vi "AndorCamera.vi"() -> ()   [LabVIEW 2018, in "AndorOWN.lvlib"]
uses:
  AndorOWN.lvlib
  Andor SDK/AndorSDK.lvlib
  SOLA/LabVIEW 2015 Library (32bit)/LumencorDLL32/LumencorDLL32.lvlib
panel:
  out "speed out":sgl
  out "fastest speed out":sgl
  out "fastest index out":i32
  out "LETypeStr out":string
  in  "ComPort":i32=5
  out "Image":T1(plugin-control)
  out "Acq. Error Array":cluster{i32, string}[](array[cluster])
  in  "Set Temperature":i32=-20
  out "Acquisition Ready?":bool
  in  "Abort Acquisition":bool
  in  "Image Name":string="TestIMG"
  in  "Camera Messages":i32(listbox)=2
  in  "Acquire Image":bool
  out "kinetic out":sgl
  out "accumulate out":sgl
  out "exposure out":sgl
  in  "Exposure Time [ms]":sgl=50.0
  in  "stop":bool
  out "Cooling Message":cluster{i32, string}
  out "Camera Temperature":sgl
  out "temperature out":sgl
  out "mintemp out":i32
  out "maxtemp out":i32
  out "AmbientTemp out":sgl
  out "TargetTemp out":sgl
  out "SensorTemp out":sgl
  out "CoolerVolts out":sgl
  out "xpixels out":i32
  out "ypixels out":i32
  out "cameraHandle out":i32
  out "totalCameras out":i32
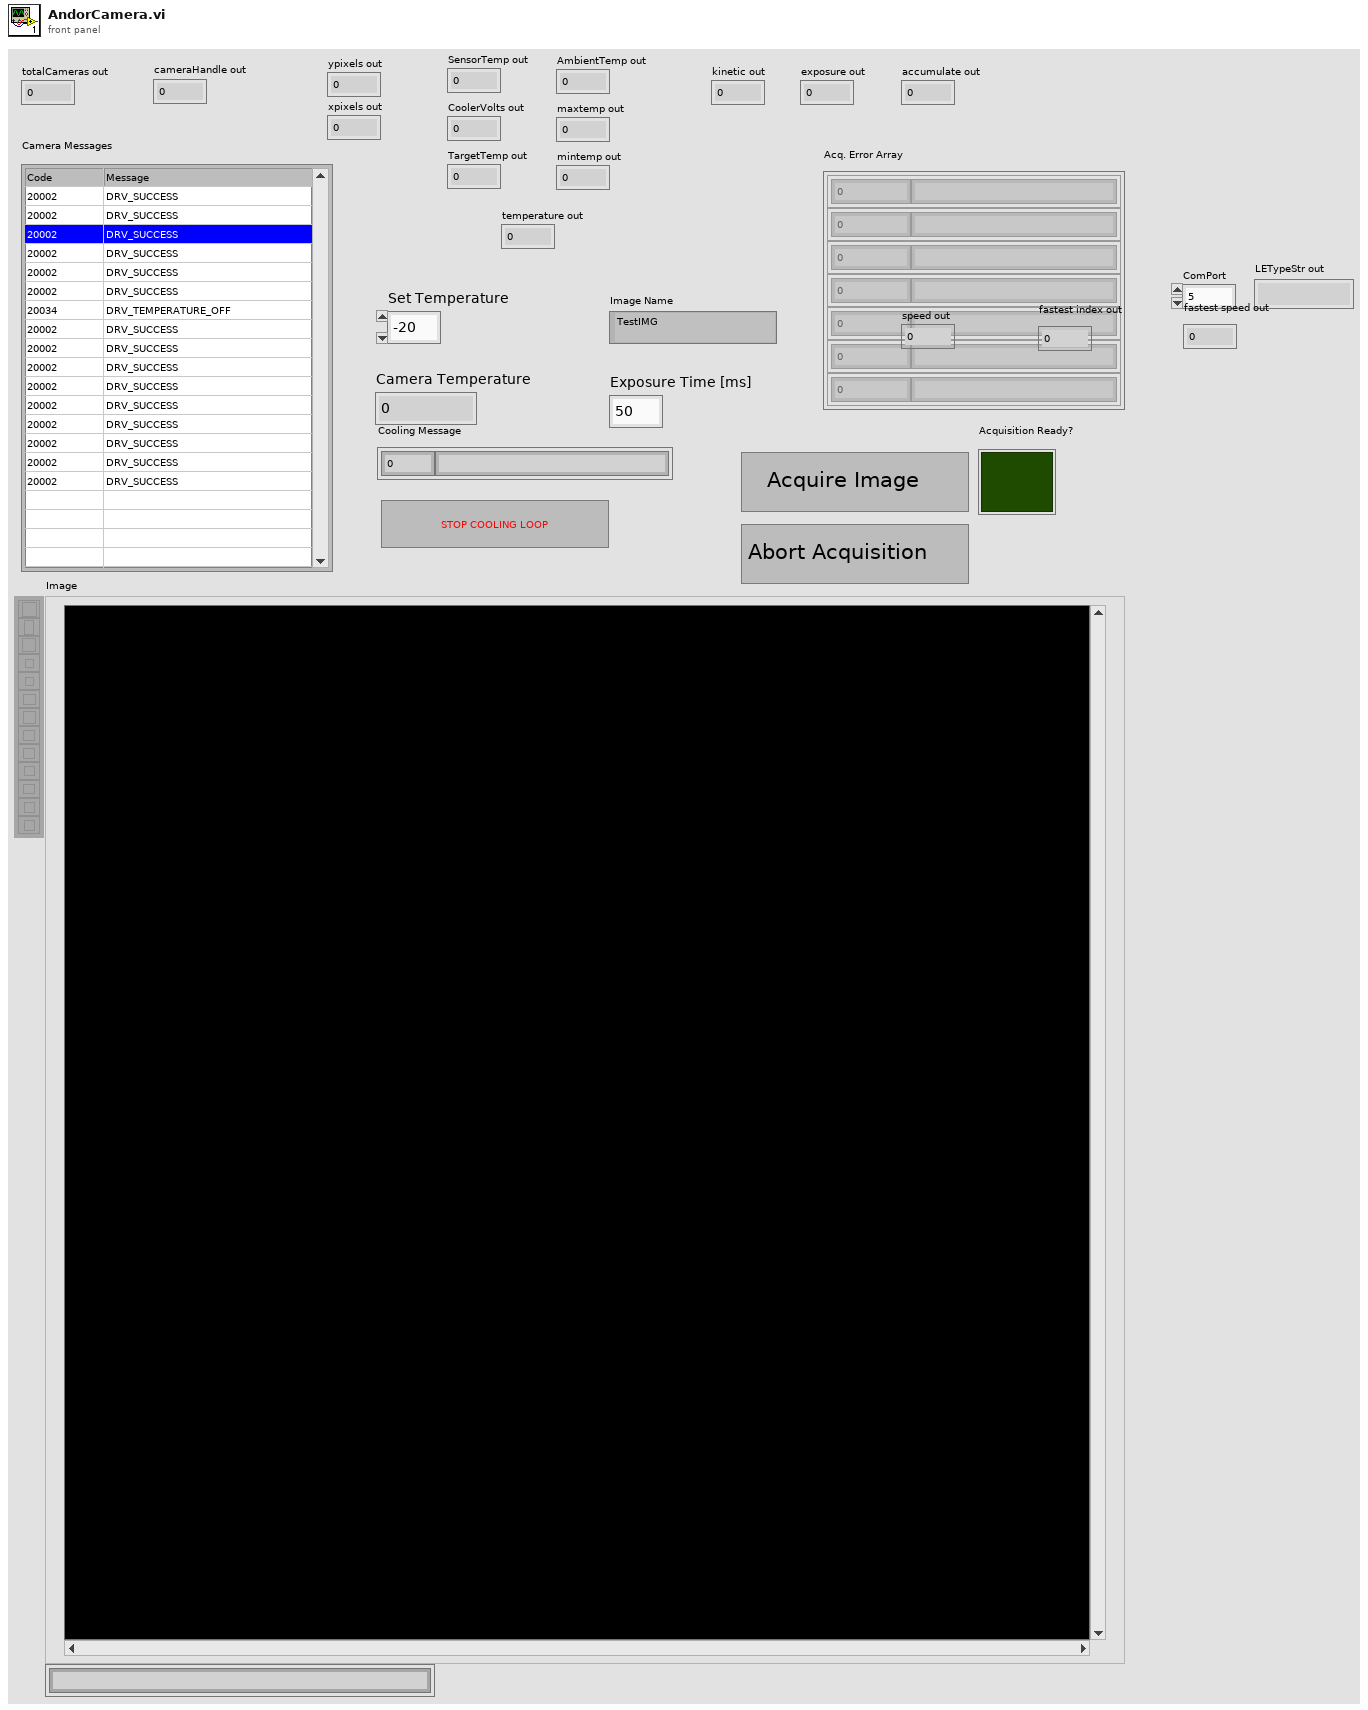
[diagram p1: front panel]
types:
  T1 = typedef "IMAQ Image.ctl" = refnum<image>
  T2 = typedef "Image Type" = u32
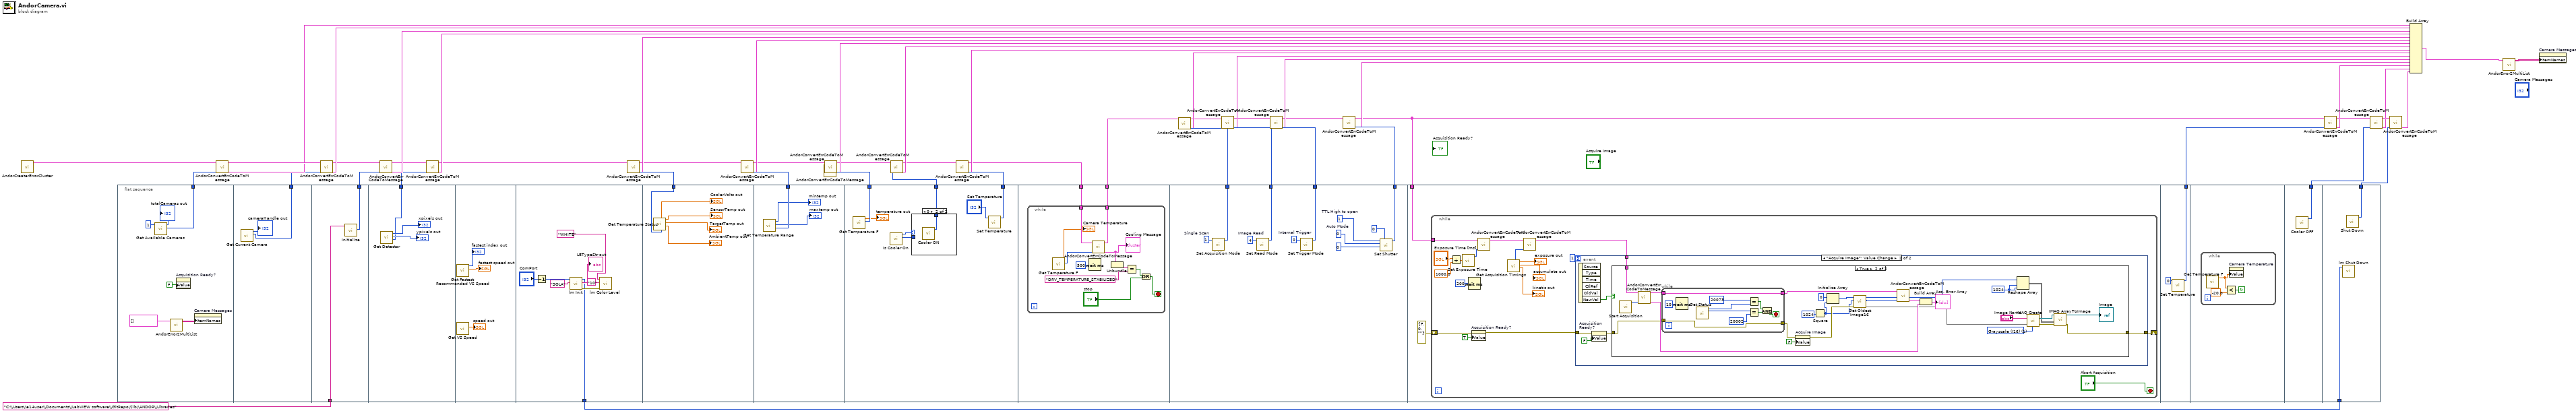
[diagram p0: block diagram]
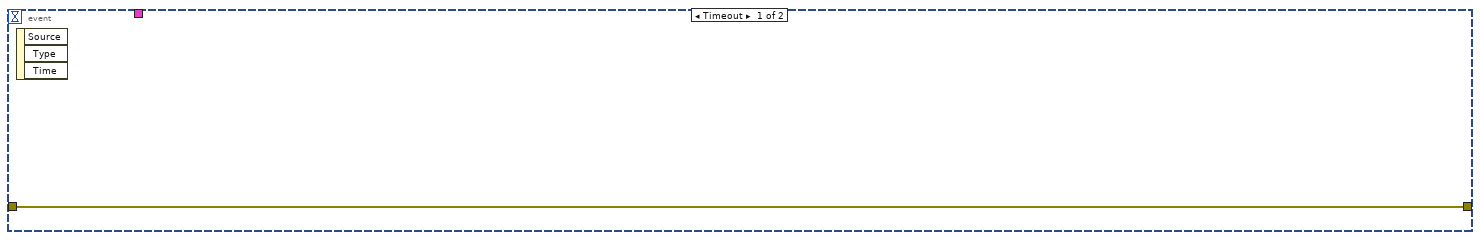
[diagram p3: hidden frame]
diagram:
  n1 = call "AndorCreaterErrorCluster.vi"() -> ("Array"=w52:cluster{i32, string}[])  [unwired: 11 in]
  n2 = flat-sequence {
    tunnel: [w57] -> w53
    tunnel: [w60] -> w44
    tunnel: "C:\\Users\\e14user\\Documents\\LabVIEW software\\GitRepo\\lib\\ANDOR\\Libraries" ("dir") -> [w63]
    tunnel: [w62] -> w42
    tunnel: [w64] -> w41
    tunnel: [w71] -> w1
    tunnel: [w82] -> w39
    tunnel: [w85] -> w37
    tunnel: [w91] -> w20
    tunnel: [w90] -> w34
    tunnel: [w87] -> w29
    tunnel: w18 -> [w96]
    tunnel: [w95] -> w17
    tunnel: [w111] -> w16
    tunnel: [w110] -> w13
    tunnel: [w109] -> w11
    tunnel: [w108] -> w8
    tunnel: w3 -> [w120]
    tunnel: [w184] -> w2
    tunnel: [w188] -> w30
    tunnel: [w190] -> w31
    tunnel: w1 -> [w189]
    frame #0 {
      n3 = call "Get Available Cameras.vi"("totalCameras"=1) -> ("function return"=w57:u32, "totalCameras out"=→"totalCameras out":i32)  [unwired: 9 in]
      n4 = call "AndorError2MultiList.vi"("Errors Messages"=cluster{i32, string}[] []) -> ("Array"=w55:string[][])  [unwired: 9 in, 1 out]
      n5 = property on="Acquisition Ready?" class="Bool (strict)"("Value"=FALSE ("Acquisition Ready?")) -> ()  [unwired: 2 in, 2 out]
      n6 = property on="Camera Messages" class="MCListbox (strict)"("ItemNames"=w55) -> ()  [unwired: 2 in, 2 out]
    }
    frame #1 {
      n7 = call "Get Current Camera.vi"() -> ("function return"=w60:u32, "cameraHandle out"=→"cameraHandle out":i32)  [unwired: 10 in]
    }
    frame #2 {
      n8 = call "Initialize.vi"("dir"=w63) -> ("function return"=w62:u32)  [unwired: 9 in, 1 out]
    }
    frame #3 {
      n9 = call "Get Detector.vi"() -> ("function return"=w64:u32, "ypixels out"=→"ypixels out":i32, "xpixels out"=→"xpixels out":i32)  [unwired: 9 in]
    }
    frame #4 {
      n10 = call "Get Fastest Recommended VS Speed.vi"() -> ("speed out"=→"fastest speed out":sgl, "index out"=→"fastest index out":i32)  [unwired: 9 in, 1 out]
      n11 = call "Get VS Speed.vi"() -> ("speed out"=→"speed out":sgl)  [unwired: 10 in, 1 out]
    }
    frame #5 {
      n12 = Decrement(x="ComPort") -> (x-1=w77:i32)
      n13 = call "lm Init.vi"("LETypeStr"="SOLA", "ComPort"=w77) -> ("error out"=w73:errorcluster, "LETypeStr out"=→"LETypeStr out":string, "function return"=w71:u32)  [unwired: 7 in]
      n14 = call "lm Color Level.vi"("error in (no error)"=w73, "str_Level"="10", "str_Color"="WHITE") -> ()  [unwired: 6 in, 3 out]
    }
    frame #6 {
      n15 = call "Get Temperature Status.vi"() -> ("AmbientTemp out"=→"AmbientTemp out":sgl, "TargetTemp out"=→"TargetTemp out":sgl, "SensorTemp out"=→"SensorTemp out":sgl, "function return"=w82:u32, "CoolerVolts out"=→"CoolerVolts out":sgl)  [unwired: 7 in]
    }
    frame #7 {
      n16 = call "Get Temperature Range.vi"() -> ("function return"=w85:u32, "maxtemp out"=→"maxtemp out":i32, "mintemp out"=→"mintemp out":i32)  [unwired: 9 in]
    }
    frame #8 {
      n17 = call "Get Temperature F.vi"() -> ("function return"=w90:u32, "temperature out"=→"temperature out":sgl)  [unwired: 10 in]
      n18 = call "Is Cooler On.vi"() -> ("function return"=w86:u32, "iCoolerStatus out"=w88:i32)  [unwired: 10 in]
      n19 = case shown="0" w88 {
        tunnel: [w93 w94] -> w87
        tunnel: w86 -> [w93 _]
        frame 1, Default {
        }
        frame 0 {
          n20 = call "Cooler ON.vi"() -> ("function return"=w94:u32)  [unwired: 11 in]
        }
      }
      n21 = call "Set Temperature.vi"("temperature"="Set Temperature") -> ("function return"=w91:u32)  [unwired: 10 in]
    }
    frame #9 {
      n22 = while {
        tunnel: w96 -> [w106]
        tunnel: [w105] -> w95
        stop <- w102 stop-if-true
        n23 = call "Get Temperature F.vi"() -> ("function return"=w107:u32, "temperature out"=→"Camera Temperature":sgl)  [unwired: 10 in]
        n24 = Wait (ms)(milliseconds to wait=u32 500) -> ()  [unwired: 1 out]
        n25 = call "AndorConvertErrCodeToMessage.vi"("function return"=w107, "Array"=w106) -> ("Element Return"=w100:cluster{i32, string}, "Array out"=w105:cluster{i32, string}[])  [unwired: 8 in]
        "Cooling Message" <- w100
        n26 = Unbundle(w100) -> (w98:string)  [unwired: 1 out]
        n27 = Equal?(x=w98, y="DRV_TEMPERATURE_STABILIZED") -> (x = y?=w99:bool)
        n28 = Or(x=w99, y="stop") -> (x .or. y?=w102:bool)
      }
    }
    frame #10 {
      w114 = 0  # Auto Mode
      w115 = 1  # TTL High to open
      w116 = 0  # Internal Trigger
      w117 = 1  # Single Scan
      w118 = 4  # Image Read
      n29 = call "Set Acquisition Mode.vi"("mode"=w117) -> ("function return"=w111:u32)  [unwired: 10 in]
      n30 = call "Set Read Mode.vi"("mode"=w118) -> ("function return"=w110:u32)  [unwired: 10 in]
      n31 = call "Set Trigger Mode.vi"("mode"=w116) -> ("function return"=w109:u32)  [unwired: 10 in]
      n32 = call "Set Shutter.vi"("openingtime"=0, "closingtime"=0, "mode"=w114, "typ"=w115) -> ("function return"=w108:u32)  [unwired: 7 in]
    }
    frame #11 {
      n33 = while {
        tunnel: w120 -> [w132]
        shift-right: [w127] -> _
        shift-left: errorcluster {"status"=FALSE, "code"=0, "source"=""} ("error in (no error)") -> [w125]
        stop <- "Abort Acquisition" stop-if-true
        n34 = Divide(x="Exposure Time [ms]", y=sgl 1000.0) -> (x/y=w122:sgl)
        n35 = call "Set Exposure Time.vi"("time"=w122) -> ("function return"=w133:u32)  [unwired: 10 in]
        n36 = Wait (ms)(milliseconds to wait=u32 200) -> ()  [unwired: 1 out]
        n37 = property on="Acquisition Ready?" class="Bool (strict)"(error in=w125, "Value"=TRUE ("Acquisition Ready?")) -> (error out=w124:errorcluster)  [unwired: 1 in, 1 out]
        n38 = call "AndorConvertErrCodeToMessage.vi"("function return"=w133, "Array"=w132) -> ("Array out"=w130:cluster{i32, string}[])  [unwired: 8 in, 1 out]
        n39 = call "Get Acquisition Timings.vi"() -> ("kinetic out"=→"kinetic out":sgl, "accumulate out"=→"accumulate out":sgl, "exposure out"=→"exposure out":sgl, "function return"=w131:u32)  [unwired: 8 in]
        n40 = call "AndorConvertErrCodeToMessage.vi"("function return"=w131, "Array"=w130) -> ("Array out"=w129:cluster{i32, string}[])  [unwired: 8 in, 1 out]
        n41 = event shown="[1] \"Acquire Image\": Value Change" {
          selector: _ -> [_ _]
          dyn-events: _ -> [_ _]
          timeout: 1 -> [_ _]
          tunnel: w129 -> [_ w144]
          tunnel: [w139 w143] -> w127
          tunnel: w124 -> [w139 w141]
          event Timeout {
            n42 = event-data() -> ()  [unwired: 1 in, 3 out]
          }
          event "Acquire Image": Value Change {
            n43 = event-data() -> ("NewVal"=w145:bool)  [unwired: 1 in, 5 out]
            n44 = property on="Acquisition \nReady?" class="Bool (strict)"(error in=w141, "Value"=FALSE ("Acquisition Ready?")) -> (error out=w140:errorcluster)  [unwired: 1 in, 1 out]
            n45 = case shown="True" w145 {
              tunnel: w144 -> [_ w170]
              tunnel: w140 -> [w146 w163]
              tunnel: [w146 w148] -> w143
              frame False {
              }
              frame True {
                w156 = T2 1 items=["Grayscale (U8)", "Grayscale (I16)", "Grayscale (SGL)", "Complex (CSG)", "RGB (U32)", "HSL (U32)", "RGB (U64)", "Grayscale (U16)"] ("Image Type")
                w157 = 1024 ("dimension size")
                n46 = call "Start Acquisition.vi"() -> ("function return"=w171:u32)  [unwired: 11 in]
                n47 = call "AndorConvertErrCodeToMessage.vi"("function return"=w171, "Array"=w170) -> ("Element Return"=w164:cluster{i32, string}, "Array out"=w169:cluster{i32, string}[])  [unwired: 8 in]
                n48 = while {
                  tunnel: w163 -> [w173]
                  tunnel: [w173] -> w162
                  tunnel: w169 -> [w174]
                  tunnel: [w174] -> w166
                  stop <- w176 stop-if-true
                  n49 = Wait (ms)(milliseconds to wait=u32 10) -> ()  [unwired: 1 out]
                  n50 = call "Get Status.vi"() -> ("function return"=w182:u32, "status out"=w179:i32)  [unwired: 10 in]
                  n51 = Equal?(x=20073 ("status out"), y=w179) -> (x = y?=w178:bool)
                  n52 = Equal?(x=w182, y=20002 ("x")) -> (x = y?=w177:bool)
                  n53 = And(x=w178, y=w177) -> (x .and. y?=w176:bool)
                }
                n54 = property on="Acquire Image" class="Bool (strict)"(error in=w162, "Value"=FALSE ("Acquire Image")) -> (error out=w160:errorcluster)  [unwired: 1 in, 1 out]
                n55 = Square(x=1024) -> (x^2=w158:i32)
                n56 = Initialize Array(0 ("element"), w158) -> (w161:i32[])
                n57 = call "Get Oldest Image16.vi"(8:w160, "size"=w158, "arr"=w161) -> (0:w151, "function return"=w159:u32, "arr out"=w152:u16)  [unwired: 6 in]
                n58 = call "AndorConvertErrCodeToMessage.vi"("function return"=w159, "Array"=w166) -> ("Element Return"=w165:cluster{i32, string})  [unwired: 8 in, 1 out]
                n59 = Build Array(w165, w164) -> (→"Acq. Error Array":cluster{i32, string}[])
                n60 = Reshape Array(w152, w157, w157) -> (w147:void[][])
                n61 = call "IMAQ Create"("Image Name"="Image Name", "Image Type"=w156, "error in (no error)"=w151) -> ("New Image"=w155:T1, "error out"=w154:errorcluster)  [unwired: 2 in]
                n62 = call "IMAQ ArrayToImage"("error in (no error)"=w154, "Image Pixels (I16)"=w147, "Image"=w155) -> ("error out"=w148:errorcluster, "Image Out"=→"Image":T1)  [unwired: 7 in]
              }
            }
          }
        }
      }
    }
    frame #12 {
      n63 = call "Set Temperature.vi"("temperature"=0) -> ("function return"=w184:u32)  [unwired: 10 in]
    }
    frame #13 {
      n64 = while {
        stop <- w186 continue-if-true
        n65 = call "Get Temperature F.vi"() -> ("temperature out"=w185:sgl)  [unwired: 10 in, 1 out]
        n66 = Less?(x=w185, y=sgl -20.0) -> (x < y?=w186:bool)
        n67 = property on="Camera Temperature" class="DigNum (strict)"("Value"=w185) -> ()  [unwired: 2 in, 2 out]
      }
    }
    frame #14 {
      n68 = call "Cooler OFF.vi"() -> ("function return"=w188:u32)  [unwired: 11 in]
    }
    frame #15 {
      n69 = call "lm Shut Down.vi"("hSerial"=w189) -> ()  [unwired: 9 in, 2 out]
      n70 = call "Shut Down.vi"() -> ("function return"=w190:u32)  [unwired: 11 in]
    }
  }
  n71 = call "AndorConvertErrCodeToMessage.vi"("function return"=w53, "Array"=w52) -> ("Element Return"=w48:cluster{i32, string}, "Array out"=w49:cluster{i32, string}[])  [unwired: 8 in]
  n72 = call "AndorConvertErrCodeToMessage.vi"("function return"=w44, "Array"=w49) -> ("Element Return"=w51:cluster{i32, string}, "Array out"=w45:cluster{i32, string}[])  [unwired: 8 in]
  n73 = call "AndorConvertErrCodeToMessage.vi"("function return"=w42, "Array"=w45) -> ("Element Return"=w47:cluster{i32, string}, "Array out"=w46:cluster{i32, string}[])  [unwired: 8 in]
  n74 = call "AndorConvertErrCodeToMessage.vi"("function return"=w41, "Array"=w46) -> ("Element Return"=w50:cluster{i32, string}, "Array out"=w40:cluster{i32, string}[])  [unwired: 8 in]
  n75 = call "AndorConvertErrCodeToMessage.vi"("function return"=w39, "Array"=w40) -> ("Element Return"=w38:cluster{i32, string}, "Array out"=w35:cluster{i32, string}[])  [unwired: 8 in]
  n76 = call "AndorConvertErrCodeToMessage.vi"("function return"=w37, "Array"=w35) -> ("Element Return"=w36:cluster{i32, string}, "Array out"=w33:cluster{i32, string}[])  [unwired: 8 in]
  n77 = call "AndorConvertErrCodeToMessage.vi"() -> ()  [unwired: 10 in, 2 out]
  n78 = call "AndorConvertErrCodeToMessage.vi"("function return"=w34, "Array"=w33) -> ("Element Return"=w32:cluster{i32, string}, "Array out"=w28:cluster{i32, string}[])  [unwired: 8 in]
  n79 = call "AndorConvertErrCodeToMessage.vi"("function return"=w29, "Array"=w28) -> ("Element Return"=w22:cluster{i32, string}, "Array out"=w21:cluster{i32, string}[])  [unwired: 8 in]
  n80 = call "AndorConvertErrCodeToMessage.vi"("function return"=w20, "Array"=w21) -> ("Element Return"=w19:cluster{i32, string}, "Array out"=w18:cluster{i32, string}[])  [unwired: 8 in]
  n81 = call "AndorConvertErrCodeToMessage.vi"("function return"=w16, "Array"=w17) -> ("Element Return"=w15:cluster{i32, string}, "Array out"=w14:cluster{i32, string}[])  [unwired: 8 in]
  n82 = call "AndorConvertErrCodeToMessage.vi"("function return"=w13, "Array"=w14) -> ("Element Return"=w10:cluster{i32, string}, "Array out"=w12:cluster{i32, string}[])  [unwired: 8 in]
  n83 = call "AndorConvertErrCodeToMessage.vi"("function return"=w11, "Array"=w12) -> ("Element Return"=w9:cluster{i32, string}, "Array out"=w7:cluster{i32, string}[])  [unwired: 8 in]
  n84 = call "AndorConvertErrCodeToMessage.vi"("function return"=w8, "Array"=w7) -> ("Element Return"=w6:cluster{i32, string}, "Array out"=w3:cluster{i32, string}[])  [unwired: 8 in]
  n85 = call "AndorConvertErrCodeToMessage.vi"("function return"=w2, "Array"=w3) -> ("Element Return"=w23:cluster{i32, string}, "Array out"=w27:cluster{i32, string}[])  [unwired: 8 in]
  n86 = call "AndorConvertErrCodeToMessage.vi"("function return"=w30, "Array"=w27) -> ("Element Return"=w24:cluster{i32, string}, "Array out"=w26:cluster{i32, string}[])  [unwired: 8 in]
  n87 = call "AndorConvertErrCodeToMessage.vi"("function return"=w31, "Array"=w26) -> ("Element Return"=w25:cluster{i32, string})  [unwired: 8 in, 1 out]
  n88 = Build Array(w48, w51, w47, w50, w38, w36, w32, w22, w19, w15, w10, w9, w6, w23, w24, w25) -> (w5:cluster{i32, string}[])
  n89 = call "AndorError2MultiList.vi"("Errors Messages"=w5) -> ("Array"=w4:string[][])  [unwired: 9 in, 1 out]
  n90 = property on="Camera Messages" class="MCListbox (strict)"("ItemNames"=w4) -> ()  [unwired: 2 in, 2 out]
